vi "programa5.vi"() -> ()   [LabVIEW 2011]
panel:
  out "Numero de Personas":i32
  out "A/C":bool
  out "Temperatura":i32(slide) scale=0.0..60.0
  in  "Seleccionar Local":u16(ring) items=["Local 1", "Local 2", "Local 3"]
  # "Debemos seleccionar el local, luego \ngenerar el numero de personas entre\n1-50 y la temperatura entre 1-60.\nEl A/C se enciende de acuerdo a los \nsiguientes casos:\n\nLocal             Condicion para encender el A/C\nLocal1        Si la temperatura es mayor a 25 o el numerode empleados es mayor a 30.\nLocal2        Si la temperatura es mayor a 28 o el numerode empleados es mayor a 32.\nLocal3        Si la temperatura es mayor a 24 o el numerode empleados es mayor a 20."
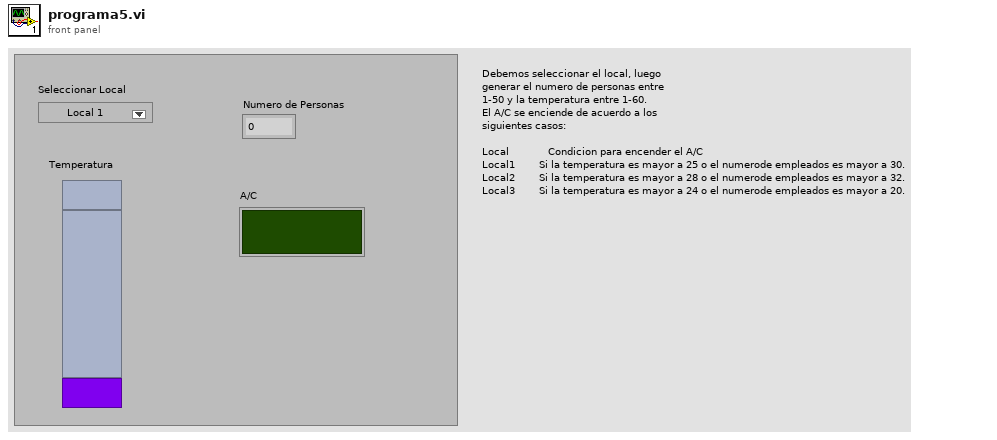
[diagram p1: front panel]
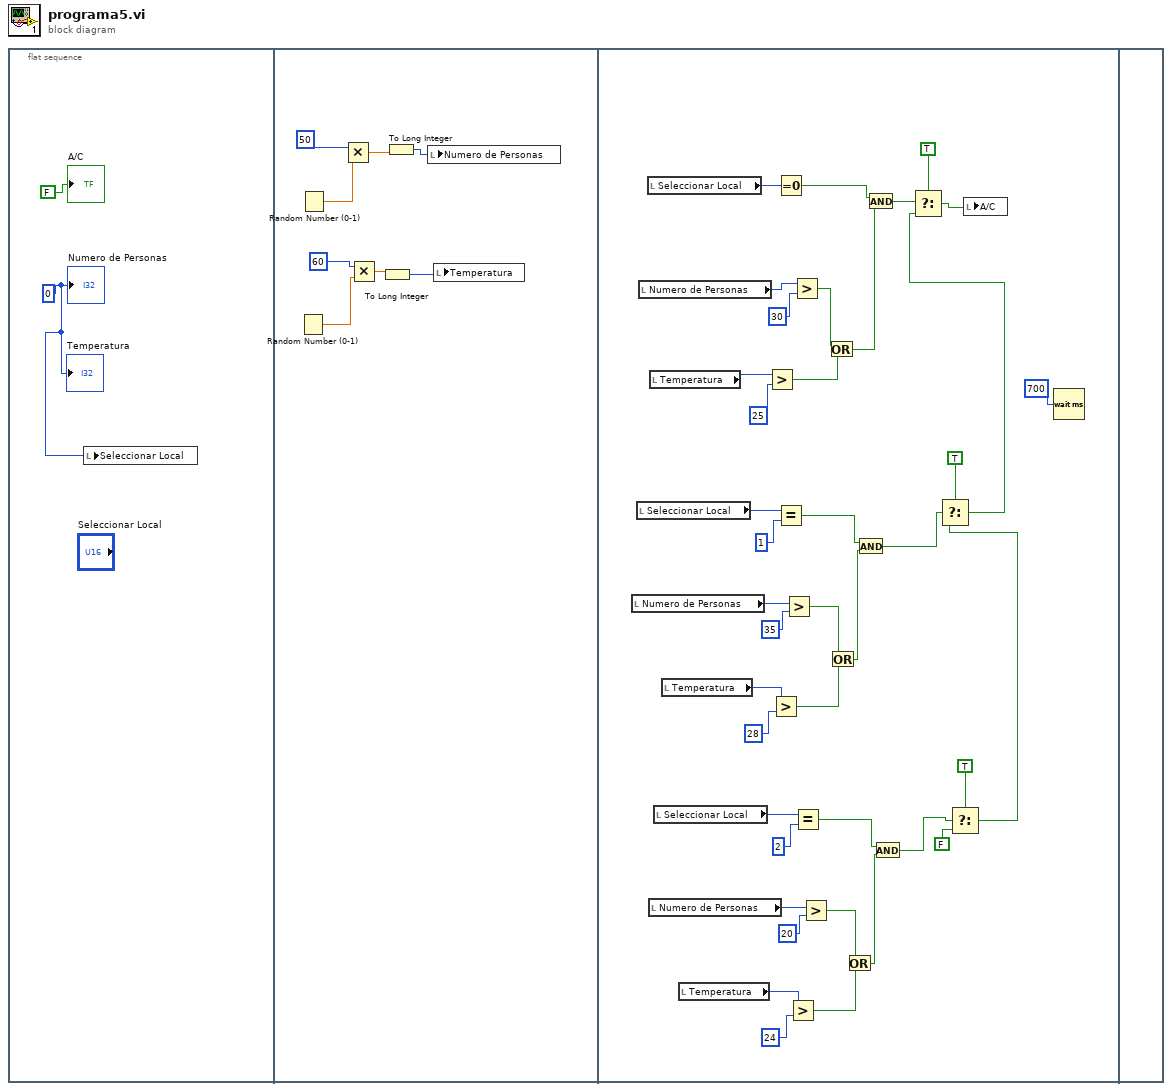
[diagram p0: block diagram]
diagram:
  n1 = flat-sequence {
    frame #0 {
      w1 = 0
      n2 = local write "Seleccionar Local"(w1) -> ()
      "Temperatura" <- w1
      "A/C" <- FALSE
      "Numero de Personas" <- w1
    }
    frame #1 {
      n3 = Random Number (0-1)() -> (number: 0 to 1=w5:dbl)
      n4 = Random Number (0-1)() -> (number: 0 to 1=w10:dbl)
      n5 = Multiply(x=50, y=w10) -> (x*y=w8:dbl)
      n6 = Multiply(x=60, y=w5) -> (x*y=w4:dbl)
      n7 = To Long Integer(number=w4) -> (32bit integer=w3:i32)
      n8 = To Long Integer(number=w8) -> (32bit integer=w7:i32)
      n9 = local write "Numero de Personas"(w7) -> ()
      n10 = local write "Temperatura"(w3) -> ()
    }
    frame #2 {
      n11 = local read "Numero de Personas"() -> (w36:i32)
      n12 = local read "Seleccionar Local"() -> (w38:u16)
      n13 = local read "Numero de Personas"() -> (w49:i32)
      n14 = local read "Seleccionar Local"() -> (w50:u16)
      n15 = local read "Numero de Personas"() -> (w19:i32)
      n16 = local read "Temperatura"() -> (w47:i32)
      n17 = local read "Seleccionar Local"() -> (w17:u16)
      n18 = local read "Temperatura"() -> (w33:i32)
      n19 = local read "Temperatura"() -> (w21:i32)
      n20 = Greater?(x=w47, y=25) -> (0:w44:bool)
      n21 = Greater?(x=w33, y=u16 28) -> (0:w31:bool)
      n22 = Equal To 0?(x=w50) -> (x = 0?=w43:bool)
      n23 = Equal?(x=w38, y=u16 1) -> (x = y?=w30:bool)
      n24 = Greater?(x=w36, y=35) -> (0:w32:bool)
      n25 = Greater?(x=w21, y=u16 24) -> (0:w23:bool)
      n26 = Greater?(x=w49, y=30) -> (0:w45:bool)
      n27 = Equal?(x=w17, y=u16 2) -> (x = y?=w24:bool)
      n28 = Greater?(x=w19, y=20) -> (0:w22:bool)
      n29 = Or(x=w45, y=w44) -> (x .or. y?=w42:bool)
      n30 = Or(x=w32, y=w31) -> (x .or. y?=w29:bool)
      n31 = Or(x=w22, y=w23) -> (x .or. y?=w25:bool)
      n32 = And(x=w30, y=w29) -> (x .and. y?=w27:bool)
      n33 = And(x=w43, y=w42) -> (x .and. y?=w41:bool)
      n34 = And(x=w24, y=w25) -> (x .and. y?=w14:bool)
      n35 = Select(t=TRUE, s=w14, f=FALSE) -> (s? t:f=w16:bool)
      n36 = Select(t=TRUE, s=w27, f=w16) -> (s? t:f=w26:bool)
      n37 = Select(t=TRUE, s=w41, f=w26) -> (s? t:f=w39:bool)
      n38 = local write "A/C"(w39) -> ()
      n39 = Wait (ms)(milliseconds to wait=700) -> ()  [unwired: 1 out]
    }
    frame #3 {
    }
  }
